vi "Apply Configuration.vi"(8 "Error In":errorcluster, 11 "reference in":refnum<class "DBC Communicator.lvclass">) -> (0 "Error Out":errorcluster, 3 "reference out":refnum<class "DBC Communicator.lvclass">)   [LabVIEW 2025, in "DBC Communicator.lvclass"]
uses:
  DBC Communicator.lvclass
  5f59e4c4-dcbf-4dc9-9909-50b1bafe8cea.vi
  5f59e4c4-dcbf-4dc9-9909-50b1bafe8cea.vi/a4169a97-72fc-4003-a778-603cf20cafa0.vi
  <vilib>/JDP Science/JSONtext/Find Item.vi
  <vilib>/JDP Science/JSONtext/Next JSON Value.vi
  <vilib>/JDP Science/JSONtext/String Subset.vi
  <vilib>/JDP Science/JSONtext/Parsing/Advance past next JSON Value (inlined COPY).vi
  <vilib>/JDP Science/JSONtext/Parsing/Advance past whitespace.vi
  <vilib>/JDP Science/JSONtext/Parsing/Advance past String.vi
  <vilib>/JDP Science/JSONtext/Parsing/Advance past Number.vi
  <vilib>/JDP Science/JSONtext/Parsing/Advance past Line Ending.vi
  <vilib>/JDP Science/JSONtext/Is Empty.vi
  <vilib>/JDP Science/JSONtext/Parsing/Parse Full Path or Item Name.vi
  <vilib>/JDP Science/JSONtext/Parsing/Advance past Array.vi
  <vilib>/JDP Science/JSONtext/Parsing/Advance past Object.vi
  <vilib>/JDP Science/JSONtext/support/Error Cluster From Code.vi
  <vilib>/JDP Science/JSONtext/Offset/Find Item Locations by Path.vi
  <vilib>/JDP Science/JSONtext/JSON text to Variant.vi
  Common-LabVIEW-Helpers/Source/errors/-8301 Item not found in JSON--error.vi
  Common-LabVIEW-Helpers/Source/errors/-8300 JSON empty--error.vi
  Communicator/Communicator.lvclass
  <vilib>/JDP Science/JSONtext/LVClass Serializer/JSONtext LVClass Serializer.lvclass
  Interfaces/IConfigure/IConfigure.lvclass
  Interfaces/IConfiguration/IConfiguration.lvclass
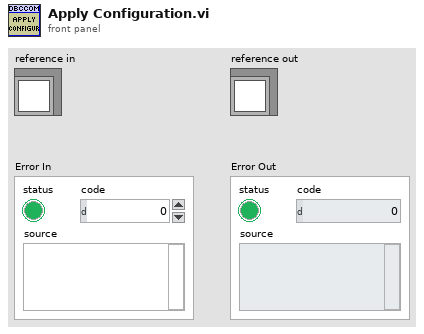
[diagram p1: front panel]
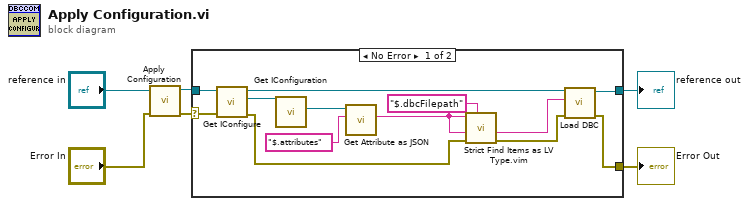
[diagram p0: block diagram]
diagram:
  n1 = call-parent "Apply Configuration.vi"("Error In"="Error In", "Communicator in"="reference in") -> ("Error Out"=w4:errorcluster, "Communicator out"=w2:refnum<class "DBC Communicator.lvclass">)  [unwired: 8 in]
  n2 = case shown="No Error" w4 {
    selector: w4 -> [w14 w20]
    tunnel: [w15 w20] -> w6
    tunnel: [w16 w21] -> w5
    tunnel: w2 -> [w13 w21]
    frame No Error {
      n3 = call-dynamic "Get IConfigure.vi"("Error In"=w14, "reference in"=w13) -> ("Error Out"=w11:errorcluster, "IConfigure"=w19:refnum<class "IConfigure.lvclass">, "reference out"=w17:refnum<class "DBC Communicator.lvclass">)  [unwired: 7 in]
      n4 = call-dynamic "Get IConfiguration.vi"("IConfigure in"=w19) -> ("IConfiguration"=w18:refnum<class "IConfiguration.lvclass">)  [unwired: 9 in, 1 out]
      n5 = call-dynamic "Get Attribute as JSON.vi"("Attribute"="$.attributes", "IConfiguration in"=w18) -> ("<JSON>"=w9:string)  [unwired: 7 in, 2 out]
      n6 = call "Strict Find Items as LV Type.vim"("$Path or Item Name"="$.dbcFilepath" ("Attribute"), "error in"=w11, "Data Type and Default Value"=w9, "<JSON>"=w9) -> ("error out"=w8:errorcluster, "Data out"=w7:string)  [unwired: 5 in, 1 out]
      n7 = call "Load DBC.vi"("error in"=w8, "DBC File"=w7, "DBCCommunication in"=w17) -> ("error out"=w15:errorcluster, "DBCCommunication out"=w16:refnum<class "DBC Communicator.lvclass">)  [unwired: 7 in]
    }
    frame Error {
    }
  }
  "Error Out" <- w6
  "reference out" <- w5
